vi "Data Collection 2.vi"() -> ()   [LabVIEW 2014]
uses:
  <vilib>/addons/control/pid/autopid.llb/PID autotuning parameters.ctl
  <vilib>/Platform/TimedLoop/XDataNode/timing_clust.ctl
  <vilib>/Platform/TimedLoop/XDataNode/nitl_modes.ctl
  <vilib>/Platform/TimedLoop/XDataNode/wakeup.ctl
  <vilib>/FPGAPlugInAG/myRIO-1900/niLvFpga_Open_myRIO-1900.vi
  <vilib>/rvi/interface/common/dynamic/niFpgaDynamicAddResources.vi
  <vilib>/Utility/file.llb/Write To Spreadsheet File (DBL).vi
  <vilib>/Utility/error.llb/Error Cluster From Error Code.vi
  <vilib>/rvi/errors/niLvFpgaAdjustHostInterfaceError.vi
  <vilib>/FPGAPlugInAG/Dynamic/niLvFpga_Close_Dynamic.vi
  <vilib>/addons/control/pid/autopid.llb/PID Online Autotuning (Relay Feedback).vi
  <vilib>/rvi/interface/nirviOpenFPGA/nirviOpenFPGA.xnode
  FPGA Bitfiles/Test_FPGATarget_CurrentControl_60eBuCSPTsI.lvbitx
  Current Control.vi
  <vilib>/rvi/interface/nirviReadWriteControl/nirviReadWriteControl.xnode
  <vilib>/rvi/interface/nirviCloseFPGA/nirviCloseFPGA.xnode
  <vilib>/Platform/TimedLoop/XDataNode/XDataNode.xnode
  <vilib>/Platform/TimedLoop/XDataNode/XDNodeRunTimeDep.lvlib
  <vilib>/rvi/interface/Simulation/niFpgaSimulationCallBeginRW.vi
  <vilib>/addons/control/pid/NI_PID_autopid.lvlib
  NiFpgaLv.dll
  <vilib>/ptbypt/NI_PtbyPt.lvlib
panel:
  out "SP and PV":T1(graph)
  out "PV Ziegler-Nichols Tuning":dbl(graph)
  in  "SP in:":dbl(slide)=30.8641975308642 scale=0.0..100.0 scale format="%.1f"
  in  "PID gains in":T2={"proportional gain (Kc)"=1.0, "integral time (Ti, min)"=0.01, "derivative time (Td, min)"=0.0} {"derivative time (Td, min)" format="%.3f"; "integral time (Ti, min)" format="%.3f"; "proportional gain (Kc)" format="%.3f"}
  in  "autotuning parameters":T3={"type of controller"=0, "relay cycles"=3, "relay amplitude"=1.0, "control specifications"=2, "PV noise level"=0.1} {"PV noise level" format="%.2f"; "control specifications" items=["normal", "fast", "slow"]; "relay amplitude" format="%.2f"; "type of controller" items=["P", "PI", "PID"]}
  out "PV Out:":dbl(slide)=19.583333333333336 scale=0.0..100.0 scale format="%.1f"
  out "SP Out:":dbl(slide)=30.8641975308642 scale=0.0..100.0 scale format="%.1f"
  out "output cluster":T4
  out "Status?":bool
  out "MV: Current (mA)":i32
  out "error out":errorcluster
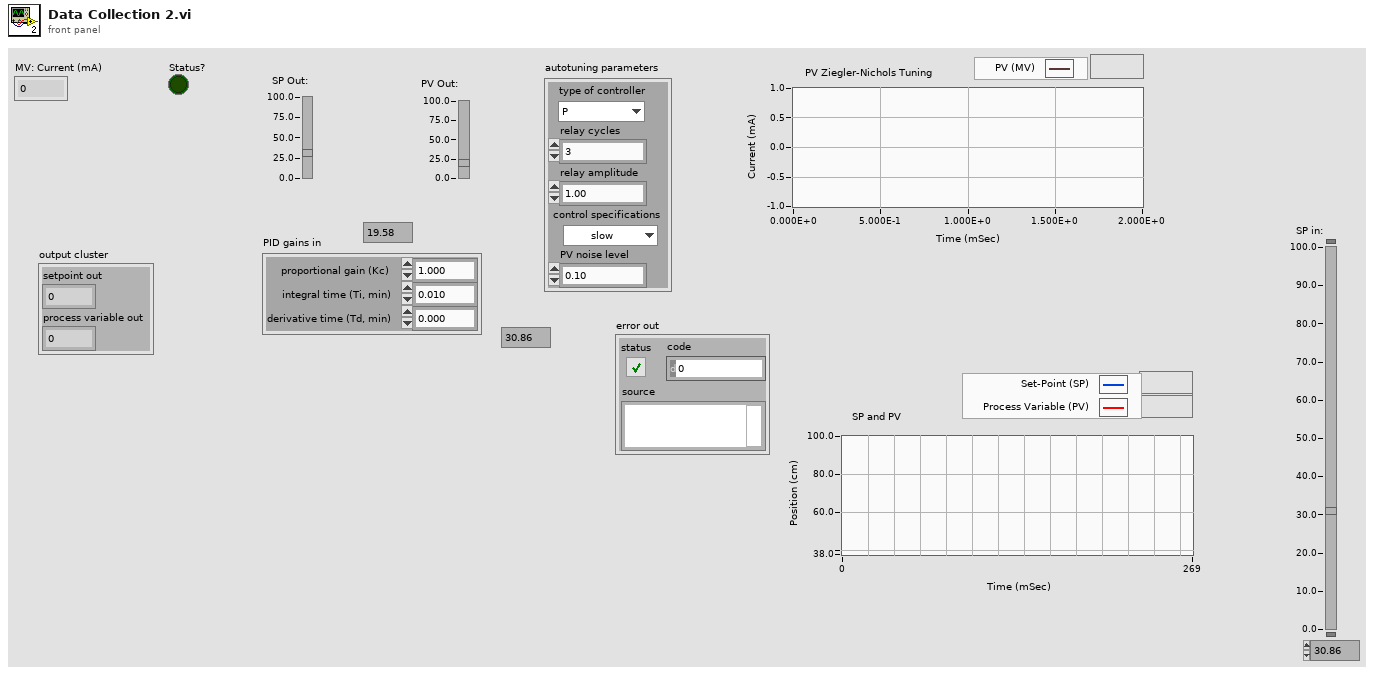
[diagram p1: front panel]
types:
  T1 = cluster{"MV: Current (mA)":i32, "PV Ziegler-Nichols Tuning":dbl}
  T2 = cluster{"proportional gain (Kc)":dbl, "integral time (Ti, min)":dbl, "derivative time (Td, min)":dbl}
  T3 = typedef "PID autotuning parameters.ctl" = cluster{"type of controller":u16, "relay cycles":i32, "relay amplitude":dbl, "control specifications":u16, "PV noise level":dbl}
  T4 = cluster{"setpoint out":dbl, "process variable out":dbl}
  T5 = typedef "XDNodeRunTimeDep.lvlib/timing_clust.ctl" = cluster{"Expected End [f-1]":u64, "Actual End [f-1]":u64, "Finished Late? [f-1]":bool, "Expected End [i-1]":u64, "Actual End [i-1]":u64, "Finished Late? [i-1]":bool, "Expected Start [i]":u64, "Actual Start [i]":u64, "Expected Start [f]":u64, "Actual Start [f]":u64, "Source Name":string, "Structure Name":string, "Period":i64, "Deadline":i64, "Offset":i64, "Start":i64, "Priority":i32, "Timeout":i32, "Mode":T6, "Wakeup Reason":T7, "Error":errorcluster, "Source Type":string, "Secondary Source Type":string, "Global End Time":u64, "Global Start Time":u64, "Frame Duration":u64, "Iteration Duration":u64, "Assigned CPU":i32, "I/O Scan Engine Mode":u32}
  T6 = typedef "XDNodeRunTimeDep.lvlib/nitl_modes.ctl" = enum32{"No Change", "Process missed periods, maintain original phase", "Discard missed periods, maintain original phase", "Process missed periods, ignore original phase", "Discard missed periods, ignore original phase"}
  T7 = typedef "XDNodeRunTimeDep.lvlib/wakeup.ctl" = enum32{"Normal", "Aborted", "Asynchronous wakeup", "Timing source error", "Timed loop error", "Timeout"}
  T8 = enum16{"big-endian, network order", "native, host order", "little-endian"}
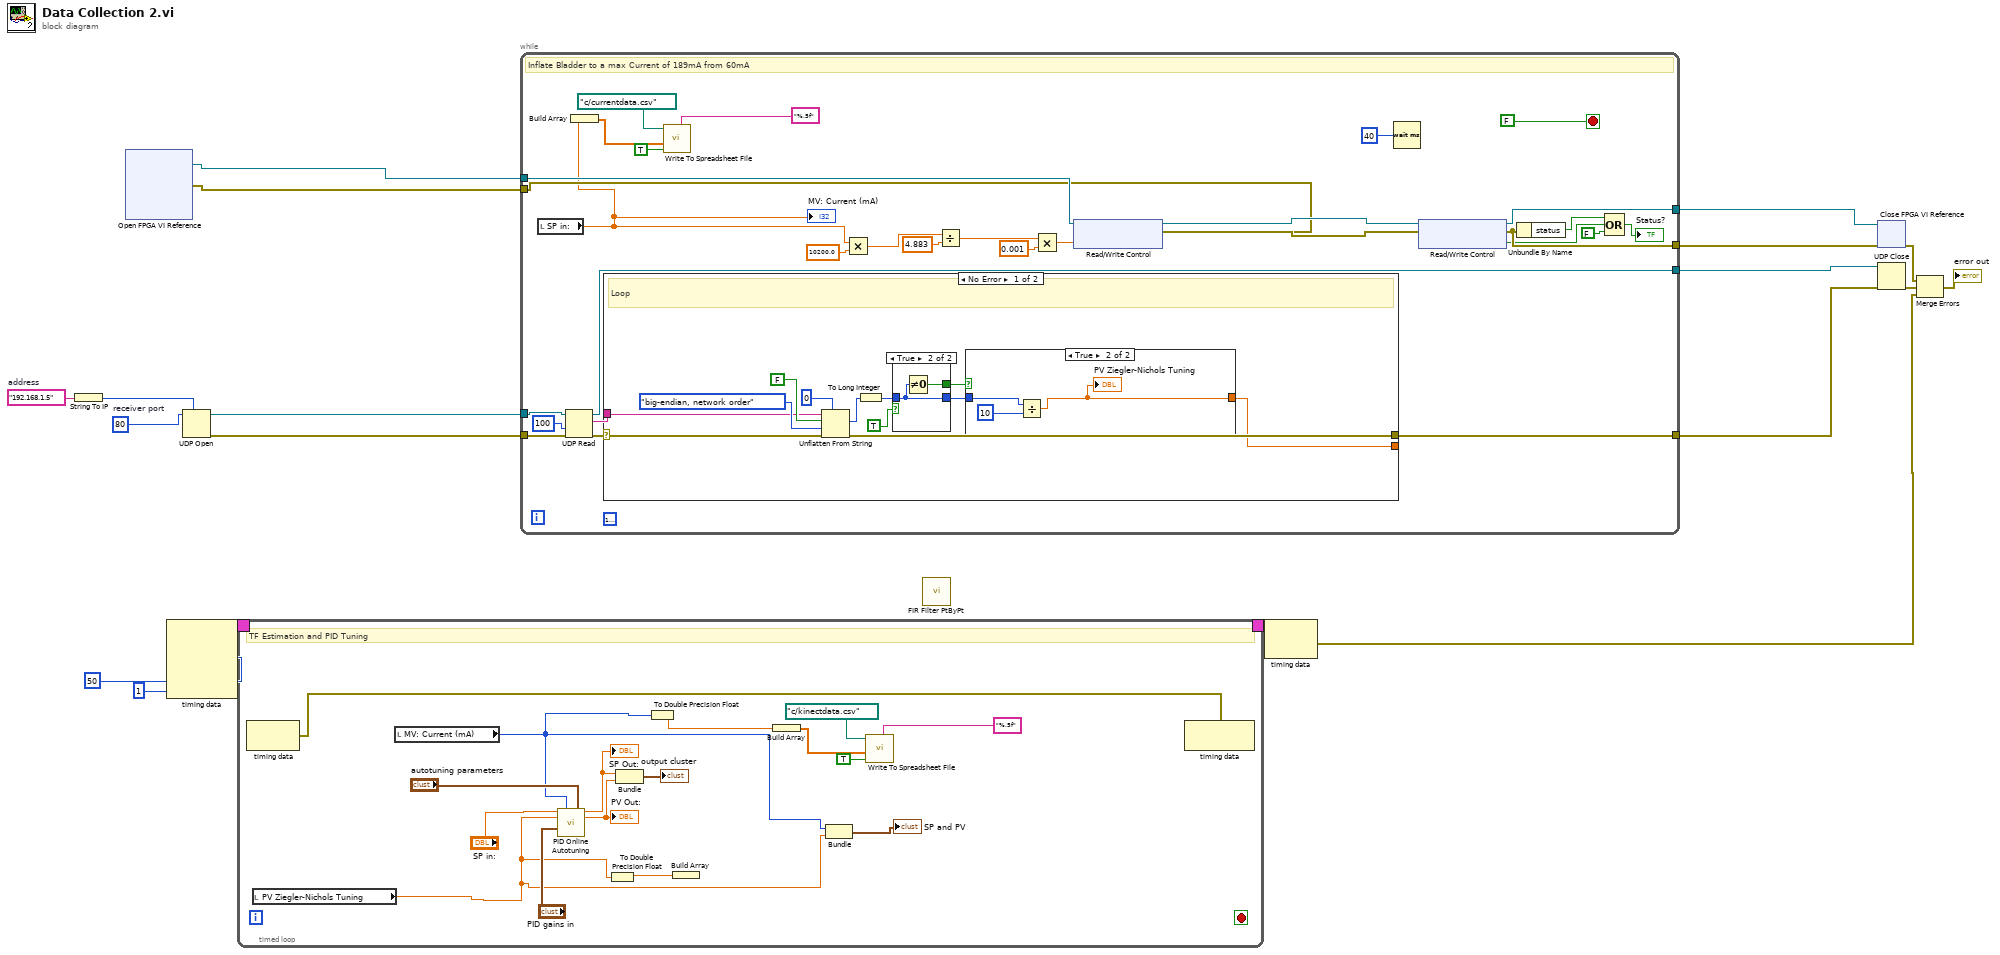
[diagram p0: block diagram]
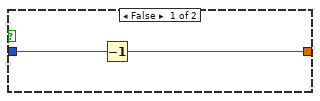
[diagram p2: hidden frame]
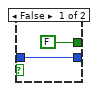
[diagram p3: hidden frame]
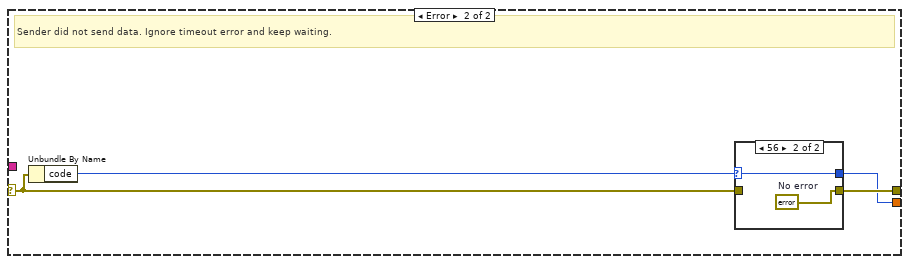
[diagram p4: hidden frame]
diagram:
  w16 = "192.168.1.5"  # address
  w15 = u16 80  # receiver port
  n1 = String To IP(1:w16) -> (0:w17:u32)
  n2 = xnode "Open FPGA VI Reference"() -> ("FPGA VI Reference Out"=w5:refnum<k20>, "error out"=w8:errorcluster)  [unwired: 2 in]
  n3 = node-c288(i64 50 ("Period"), 1 ("Processor")) -> (w19:T5)  [unwired: 2 in]
  n4 = UDP Open(7:w17, 11:w15) -> (port=w14:refnum<k16>, 0:w13:errorcluster)  [unwired: 3 in, 1 out]
  n5 = timed-loop {
    timing: w19 -> [_]
    timing-out: [_] -> w18
    stop <- _ stop-if-true
    # "TF Estimation and PID Tuning"
    n6 = node-c288() -> (w27:errorcluster)  [unwired: 1 in]
    n7 = local read "PV Ziegler-Nichols Tuning"() -> (w20:dbl)
    n8 = local read "MV: Current (mA)"() -> (w21:i32)
    n9 = call-poly <vilib>:"PID Online Autotuning.vi"("setpoint"="SP in:", "manipulated variable"=w21, "autotuning parameters"="autotuning parameters", "process variable"=w20, "PID gains in"="PID gains in") -> ("setpoint out"=w33:dbl, "process variable out"=w32:dbl)  [unwired: 6 in, 3 out]
    "PV Out:" <- w32
    "SP Out:" <- w33
    n10 = To Double Precision Float(number=w20) -> (double precision float=w29:dbl)
    n11 = Bundle("setpoint out"=w33, "process variable out"=w32) -> (→"output cluster":T4)  [unwired: 1 in]
    n12 = To Double Precision Float(number=w21) -> (double precision float=w30:dbl)
    n13 = Build Array(w29) -> ()  [unwired: 1 out]
    n14 = Build Array(w30) -> (w25:dbl[])
    n15 = Bundle("MV: Current (mA)"=w21, "PV Ziegler-Nichols Tuning"=w20) -> (→"SP and PV":T1)  [unwired: 1 in]
    n16 = call-poly <vilib>:"Write To Spreadsheet File.vi"("format (%.3f)"="%.5f", "append to file? (new file:F)"=TRUE, "1D data"=w25, "file path (dialog if empty)"=path "c:/kinectdata.csv") -> ()  [unwired: 4 in, 1 out]
    n17 = node-c288(w27) -> ()  [unwired: 1 out]
  }
  n18 = while {
    tunnel: w14 -> [w70]
    tunnel: [w68] -> w12
    tunnel: w13 -> [w69]
    tunnel: w5 -> [w64]
    tunnel: [w65] -> w6
    tunnel: w8 -> [w48]
    tunnel: [w66] -> w7
    tunnel: [w49] -> w3
    stop <- FALSE stop-if-true
    (unwired) u32 16777216
    # "Inflate Bladder to a max Current of 189mA from 60mA"
    n19 = local read "SP in:"() -> (w41:dbl)
    "MV: Current (mA)" <- w41
    n20 = UDP Read(connection ID=w70, timeout ms (25000)=100, 8:w69) -> (data out=w51:string, error out=w50:errorcluster, 3:w68:refnum<k16>)  [unwired: 3 out]
    n21 = Build Array(w41) -> (w44:dbl[])
    n22 = case shown="No Error" w50 {
      selector: w50 -> [w77 w94]
      tunnel: w51 -> [w78 _]
      tunnel: [w76 w93] -> w49
      tunnel: [w71 w92] -> _
      frame No Error {
        # "Loop"
        n23 = Unflatten From String(type=0, binary string=w78, data includes array or string size? (T)=FALSE, byte order (0:big-endian, network order)=T8."big-endian, network order" ("byte order"), error in (no error)=w77) -> (value=w79:i32, error out=w76:errorcluster)  [unwired: 1 out]
        n24 = To Long Integer(number=w79) -> (32bit integer=w74:i32)
        n25 = case shown="True" TRUE {
          tunnel: w74 -> [w88 w90]
          tunnel: [FALSE w91] -> w73
          tunnel: [w88 w90] -> w72
          frame False {
          }
          frame True {
            n26 = Not Equal To 0?(x=w90) -> (x != 0?=w91:bool)
          }
        }
        n27 = case shown="True" w73 {
          tunnel: w72 -> [w84 w86]
          tunnel: [w83 w85] -> w71
          frame False {
            n28 = Decrement(x=w84) -> (x-1=w83:i32)
          }
          frame True {
            n29 = Divide(x=w86, y=10) -> (x/y=w85:dbl)
            "PV Ziegler-Nichols Tuning" <- w85
          }
        }
      }
      frame Error {
        # "Sender did not send data. Ignore timeout error and keep waiting."
        n30 = Unbundle By Name(w94) -> ("code"=w95:i32)
        n31 = case shown="56" w95 {
          selector: w95 -> [w96 w98]
          tunnel: w94 -> [w97 _]
          tunnel: [w97 w99] -> w93
          tunnel: [w96 w98] -> w92
          frame Default {
          }
          frame 56 {
            w99 = errorcluster {"status"=FALSE, "code"=0, "source"=""}  # No error
          }
        }
      }
    }
    n32 = call-poly <vilib>:"Write To Spreadsheet File.vi"("format (%.3f)"="%.5f", "append to file? (new file:F)"=TRUE, "1D data"=w44, "file path (dialog if empty)"=path "c:/currentdata.csv") -> ()  [unwired: 4 in, 1 out]
    n33 = Multiply(x=w41, y=10200.0) -> (x*y=w52:dbl)
    n34 = Divide(x=w52, y=4.883) -> (x/y=w55:dbl)
    n35 = Multiply(x=w55, y=0.001) -> (x*y=w61:dbl)
    n36 = xnode "Read/Write Control"("FPGA VI Reference In"=w64, "error in"=w48, "DAC Inlet Valve"=w61) -> ("FPGA VI Reference Out"=w63:refnum<k20>, "error out"=w62:errorcluster)
    n37 = Wait (ms)(milliseconds to wait=u32 40) -> ()  [unwired: 1 out]
    n38 = xnode "Read/Write Control"("FPGA VI Reference In"=w63, "error in"=w62) -> ("FPGA VI Reference Out"=w65:refnum<k20>, "error out"=w66:errorcluster, "Inlet Overflow?"=w60:bool)
    n39 = Unbundle By Name(w66) -> ("status"=w58:bool)
    n40 = Compound Arithmetic op=OR(w58, w60, FALSE ("value")) -> (→"Status?":bool)
  }
  n41 = call <vilib>:"FIR Filter PtByPt.vi"() -> ()  [unwired: 4 in, 2 out]
  n42 = node-c288(w18) -> (w1:errorcluster)
  n43 = xnode "Close FPGA VI Reference"("FPGA VI Reference In"=w6, "error in"=w7) -> ("error out"=w9:errorcluster)
  n44 = UDP Close(connection ID=w12, 8:w3) -> (error out=w11:errorcluster)  [unwired: 1 out]
  n45 = Merge Errors(w9, w11, w1) -> (→"error out":errorcluster)
